vi "Data Retrieve GUI.vi"(0 "File or Folder Path":path=path "C:/", 1 "Data Type":T3=enum."DAT", 2 "DAT header length":i32=11, 5 "offset":i32, 7 "length":i32=1, 11 "error in (no error)":errorcluster) -> (4 "A vs B":cluster{dbl[], dbl[]}[](graph), 6 "C vs D":cluster{dbl[], dbl[]}[](graph), 8 "E":dbl[][](graph), 14 "Notes":string)   [LabVIEW 2019, in "LV-Data.lvclass"]
uses:
  LV-Data.lvclass
  <vilib>/Utility/miscctls.llb/LVOffsetAndMultiplierTypeDef.ctl
  LV-Data.ITX/Typedefs/Retrieve Data Type.ctl
  Typedefs/Map Variant--map.ctl
  b9190c8c-04b9-4fe6-9890-9f3313ef96ba.vi
  59021a08-4f23-4d52-b62b-93f2ba281558.vi
  LV-Data.ITX/LV-Data.ITX.lvclass
  <userlib>/LevyLab/Graph Utilities/graph_utilities.lvclass
panel:
  out "Current State":string
  in  "Update Graphs":bool
  in  "Read Files":bool
  in  "Initialize Keys":bool
  out "N":T1(array[cluster]) {"N5" format="%#_6p"; "N4" format="%#_6p"; "N3" format="%#_6p"; "N2" format="%#_6p"; "N1" format="%#_6p"}
  in  "keys":T2 {"N5" items=["AI1", "AI10", "AI11", "AI12", "AI2", "AI3", "AI4", "AI5", "AI6", "AI7", "AI8", "AI9", "AO1", "AO10", "AO11", "AO12", "AO2", "AO3", "AO4", "AO5", "AO6", "AO7", "AO8", "AO9", "Magnet", "Magnet Field", "OFF", "Temperature", "Time", "X1", "X10", "X11", "X12", "X2", "X3", "X4", "X5", "X6", "X7", "X8", "X9", "Y1", "Y10", "Y11", "Y12", "Y2", "Y3", "Y4", "Y5", "Y6", "Y7", "Y8", "Y9"]; "N4" items=["AI1", "AI10", "AI11", "AI12", "AI2", "AI3", "AI4", "AI5", "AI6", "AI7", "AI8", "AI9", "AO1", "AO10", "AO11", "AO12", "AO2", "AO3", "AO4", "AO5", "AO6", "AO7", "AO8", "AO9", "Magnet", "Magnet Field", "OFF", "Temperature", "Time", "X1", "X10", "X11", "X12", "X2", "X3", "X4", "X5", "X6", "X7", "X8", "X9", "Y1", "Y10", "Y11", "Y12", "Y2", "Y3", "Y4", "Y5", "Y6", "Y7", "Y8", "Y9"]; "N3" items=["AI1", "AI10", "AI11", "AI12", "AI2", "AI3", "AI4", "AI5", "AI6", "AI7", "AI8", "AI9", "AO1", "AO10", "AO11", "AO12", "AO2", "AO3", "AO4", "AO5", "AO6", "AO7", "AO8", "AO9", "Magnet", "Magnet Field", "OFF", "Temperature", "Time", "X1", "X10", "X11", "X12", "X2", "X3", "X4", "X5", "X6", "X7", "X8", "X9", "Y1", "Y10", "Y11", "Y12", "Y2", "Y3", "Y4", "Y5", "Y6", "Y7", "Y8", "Y9"]; "N2" items=["AI1", "AI10", "AI11", "AI12", "AI2", "AI3", "AI4", "AI5", "AI6", "AI7", "AI8", "AI9", "AO1", "AO10", "AO11", "AO12", "AO2", "AO3", "AO4", "AO5", "AO6", "AO7", "AO8", "AO9", "Magnet", "Magnet Field", "OFF", "Temperature", "Time", "X1", "X10", "X11", "X12", "X2", "X3", "X4", "X5", "X6", "X7", "X8", "X9", "Y1", "Y10", "Y11", "Y12", "Y2", "Y3", "Y4", "Y5", "Y6", "Y7", "Y8", "Y9"]; "N1" items=["AI1", "AI10", "AI11", "AI12", "AI2", "AI3", "AI4", "AI5", "AI6", "AI7", "AI8", "AI9", "AO1", "AO10", "AO11", "AO12", "AO2", "AO3", "AO4", "AO5", "AO6", "AO7", "AO8", "AO9", "Magnet", "Magnet Field", "OFF", "Temperature", "Time", "X1", "X10", "X11", "X12", "X2", "X3", "X4", "X5", "X6", "X7", "X8", "X9", "Y1", "Y10", "Y11", "Y12", "Y2", "Y3", "Y4", "Y5", "Y6", "Y7", "Y8", "Y9"]; "E" items=["AI1", "AI10", "AI11", "AI12", "AI2", "AI3", "AI4", "AI5", "AI6", "AI7", "AI8", "AI9", "AO1", "AO10", "AO11", "AO12", "AO2", "AO3", "AO4", "AO5", "AO6", "AO7", "AO8", "AO9", "Magnet", "Magnet Field", "OFF", "Temperature", "Time", "X1", "X10", "X11", "X12", "X2", "X3", "X4", "X5", "X6", "X7", "X8", "X9", "Y1", "Y10", "Y11", "Y12", "Y2", "Y3", "Y4", "Y5", "Y6", "Y7", "Y8", "Y9"]; "D" items=["AI1", "AI10", "AI11", "AI12", "AI2", "AI3", "AI4", "AI5", "AI6", "AI7", "AI8", "AI9", "AO1", "AO10", "AO11", "AO12", "AO2", "AO3", "AO4", "AO5", "AO6", "AO7", "AO8", "AO9", "Magnet", "Magnet Field", "OFF", "Temperature", "Time", "X1", "X10", "X11", "X12", "X2", "X3", "X4", "X5", "X6", "X7", "X8", "X9", "Y1", "Y10", "Y11", "Y12", "Y2", "Y3", "Y4", "Y5", "Y6", "Y7", "Y8", "Y9"]; "C" items=["AI1", "AI10", "AI11", "AI12", "AI2", "AI3", "AI4", "AI5", "AI6", "AI7", "AI8", "AI9", "AO1", "AO10", "AO11", "AO12", "AO2", "AO3", "AO4", "AO5", "AO6", "AO7", "AO8", "AO9", "Magnet", "Magnet Field", "OFF", "Temperature", "Time", "X1", "X10", "X11", "X12", "X2", "X3", "X4", "X5", "X6", "X7", "X8", "X9", "Y1", "Y10", "Y11", "Y12", "Y2", "Y3", "Y4", "Y5", "Y6", "Y7", "Y8", "Y9"]; "B" items=["AI1", "AI10", "AI11", "AI12", "AI2", "AI3", "AI4", "AI5", "AI6", "AI7", "AI8", "AI9", "AO1", "AO10", "AO11", "AO12", "AO2", "AO3", "AO4", "AO5", "AO6", "AO7", "AO8", "AO9", "Magnet", "Magnet Field", "OFF", "Temperature", "Time", "X1", "X10", "X11", "X12", "X2", "X3", "X4", "X5", "X6", "X7", "X8", "X9", "Y1", "Y10", "Y11", "Y12", "Y2", "Y3", "Y4", "Y5", "Y6", "Y7", "Y8", "Y9"]; "A" items=["AI1", "AI10", "AI11", "AI12", "AI2", "AI3", "AI4", "AI5", "AI6", "AI7", "AI8", "AI9", "AO1", "AO10", "AO11", "AO12", "AO2", "AO3", "AO4", "AO5", "AO6", "AO7", "AO8", "AO9", "Magnet", "Magnet Field", "OFF", "Temperature", "Time", "X1", "X10", "X11", "X12", "X2", "X3", "X4", "X5", "X6", "X7", "X8", "X9", "Y1", "Y10", "Y11", "Y12", "Y2", "Y3", "Y4", "Y5", "Y6", "Y7", "Y8", "Y9"]}
  in  "OK":bool
  in  "D  is time?":bool
  in  "B is time?":bool
  out "time":string[][](table)
  in  "Use Folder Index File?":bool
  in  "Generate Folder Index File?":bool
  in  "Ez name":string="Ez name"
  in  "Ey name":string="Ey name"
  in  "Ex name":string="Ex name"
  in  "C y name":string="C y name"
  in  "D x name":string="D x name"
  in  "A y name":string="A y name"
  in  "B x name":string="B x name"
  out "Index, Wavenames":string[][](table)
  in  "recolor traces?":bool
  in  "Ex":T4={"Offset"=0.0, "Multiplier"=1.0}
  in  "Ey":T4={"Offset"=0.0, "Multiplier"=1.0}
  out "counter":i32
  out "pattern":string="*.dat"
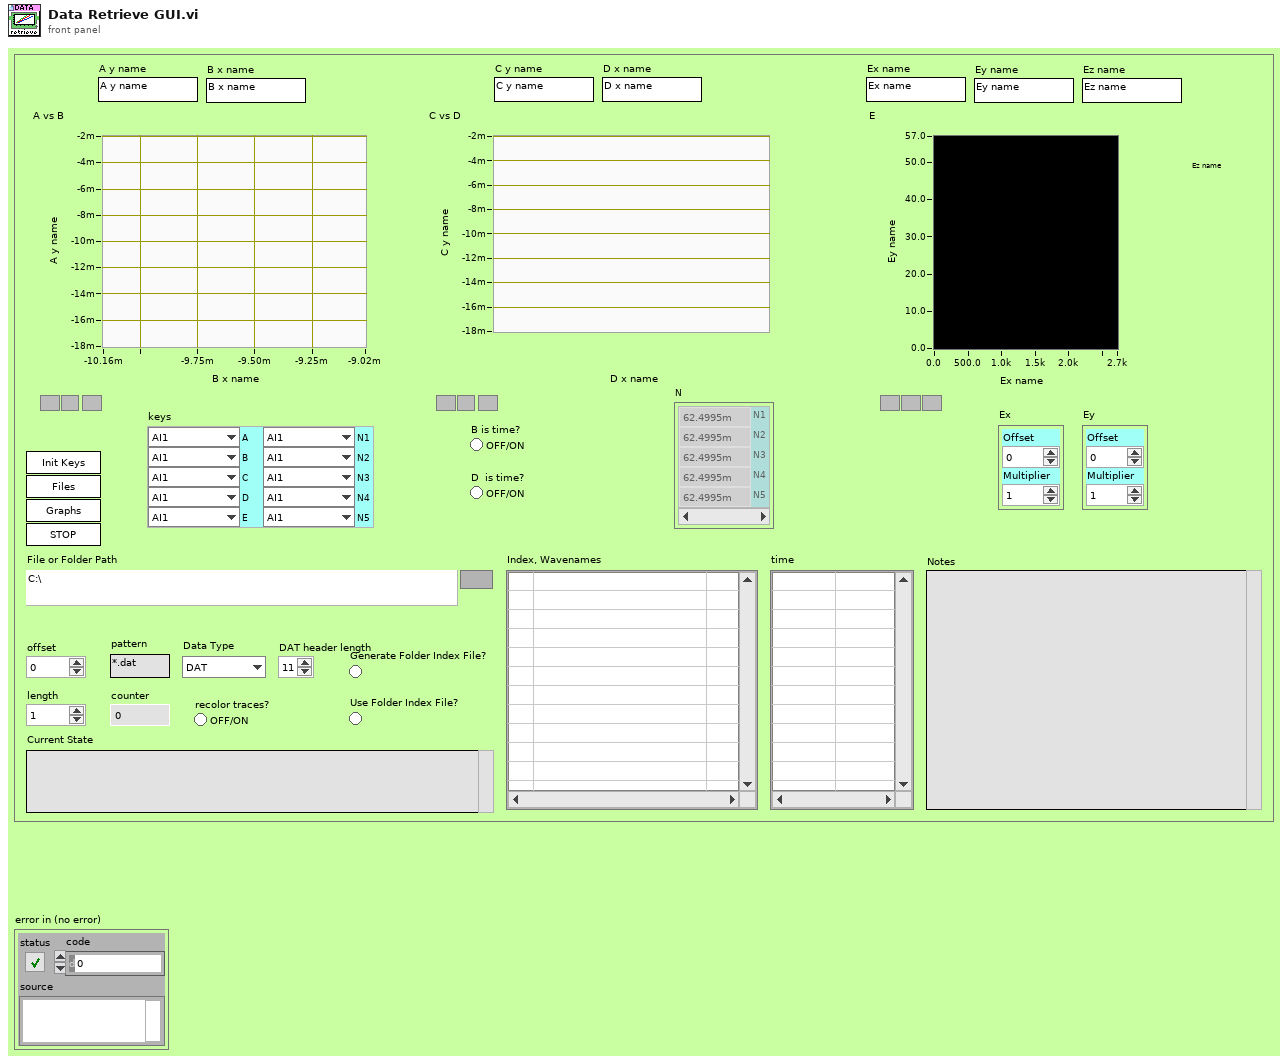
[diagram p1: front panel]
types:
  T1 = cluster{"N1":dbl, "N2":dbl, "N3":dbl, "N4":dbl, "N5":dbl}[]
  T2 = cluster{"A":u16, "B":u16, "C":u16, "D":u16, "E":u16, "N1":u16, "N2":u16, "N3":u16, "N4":u16, "N5":u16}
  T3 = typedef "LV-Data.ITX.lvclass/Retrieve Data Type.ctl" = enum16{"ITX", "ITX w/ 2D", "DAT", "TDMS"}
  T4 = typedef "LVOffsetAndMultiplierTypeDef.ctl" = cluster{"Offset":dbl, "Multiplier":dbl}
  T5 = enum32{"Invalid", "Standard", "Closed", "Hidden", "Minimized", "Maximized"}
  T6 = enum32{"invalid app kind", "Development System", "Run Time System", "Student Edition", "Embedded LabVIEW", "Evaluation", "Custom"}
  T7 = typedef "LV-Data.lvclass/Map Variant--map.ctl" = map{string, variant}
  T8 = cluster{"N1":dbl, "N2":dbl, "N3":dbl, "N4":dbl, "N5":dbl}
  T9 = cluster{"Core":cluster{"Current VI Reference":refnum<vi>, "Close Panel on Exit?":bool}, "Files":path[], "Append Index":i32, "Running Step":i32, "Data Map":T7[], "ring map":map{string, refnum<vi>}, "Wavenames":string[], "A vs B":cluster{dbl[], dbl[]}[], "C vs D":cluster{dbl[], dbl[]}[], "E":dbl[][]}
  T10 = cluster{"Current VI Reference":refnum<vi>, "Close Panel on Exit?":bool}
  T11 = typedef "LV-Data.lvclass/Dictionary--cluster.ctl" = cluster{"key":string, "value":variant}
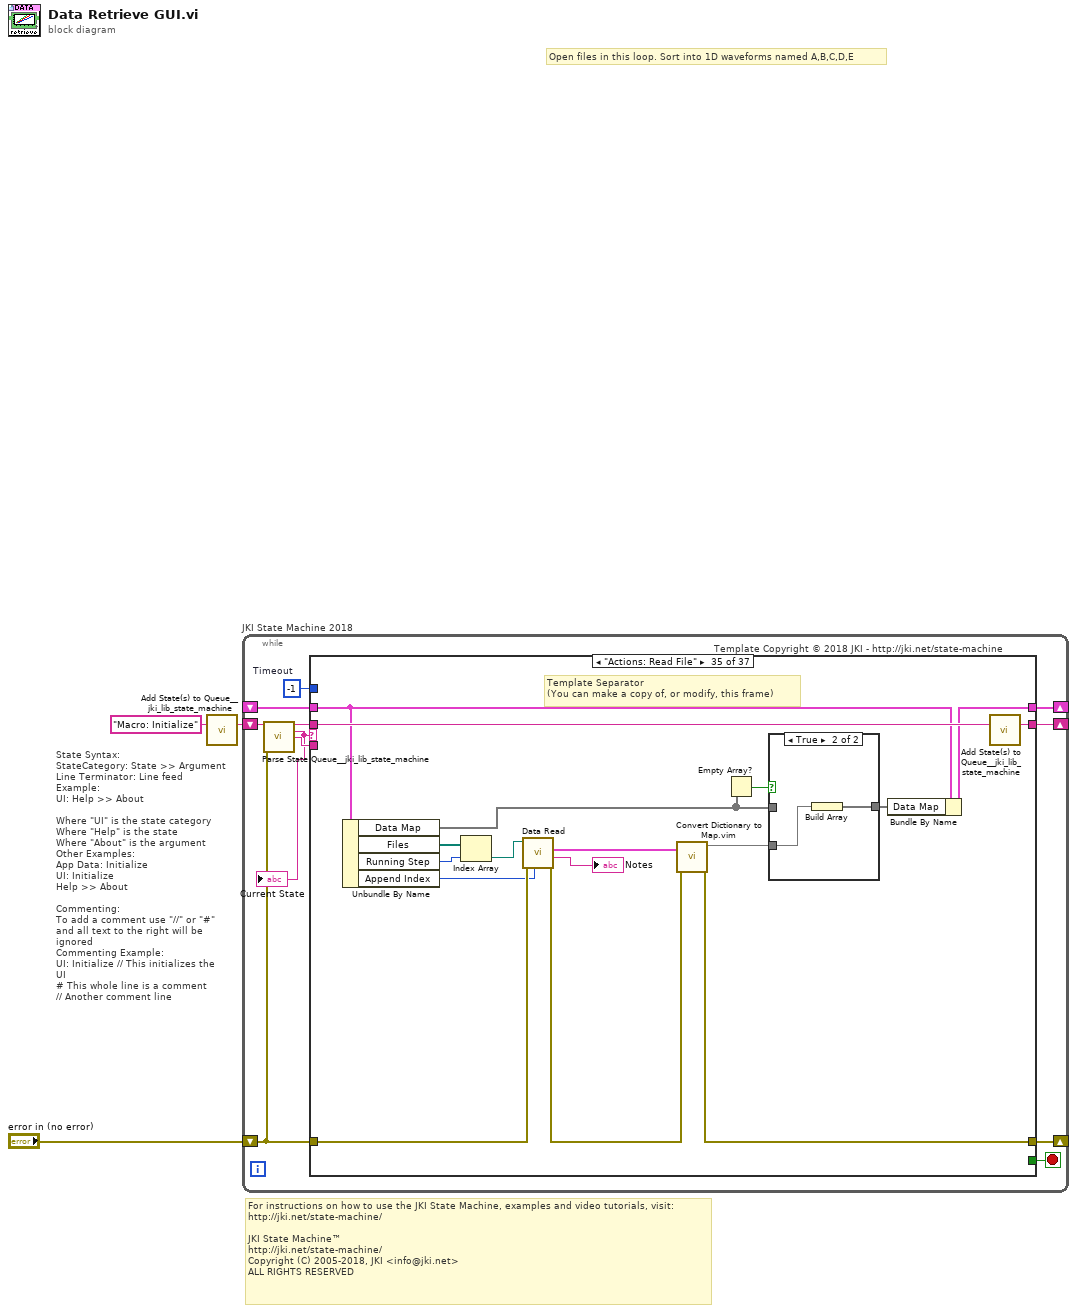
[diagram p0: block diagram]
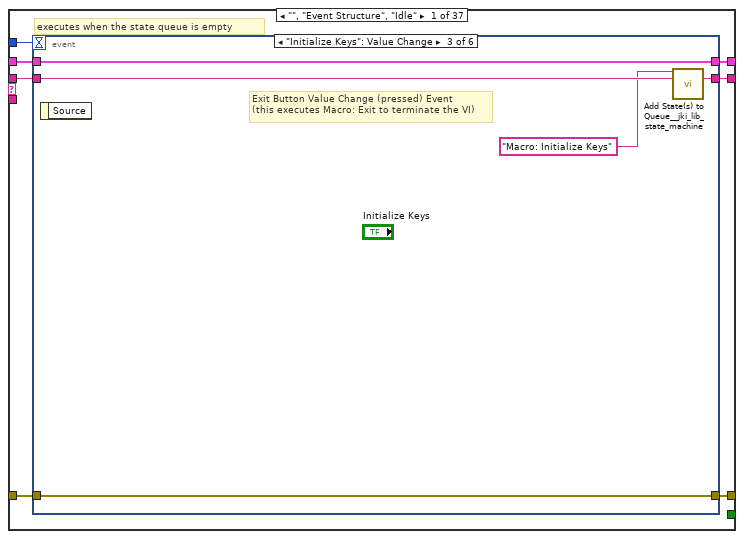
[diagram p2: hidden frame]
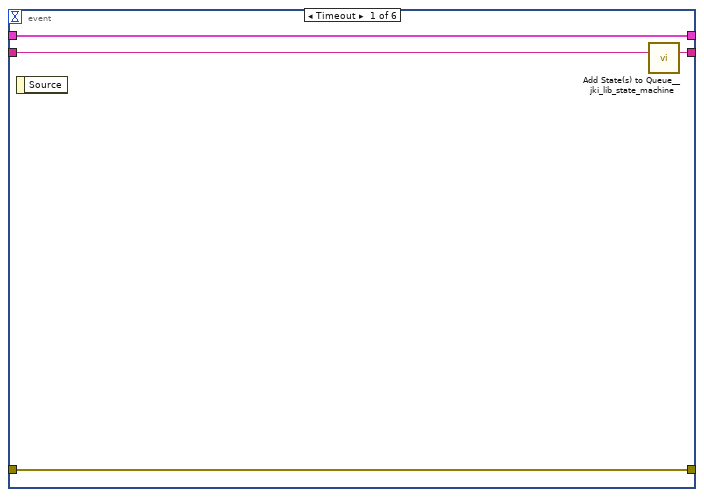
[diagram p3: hidden frame]
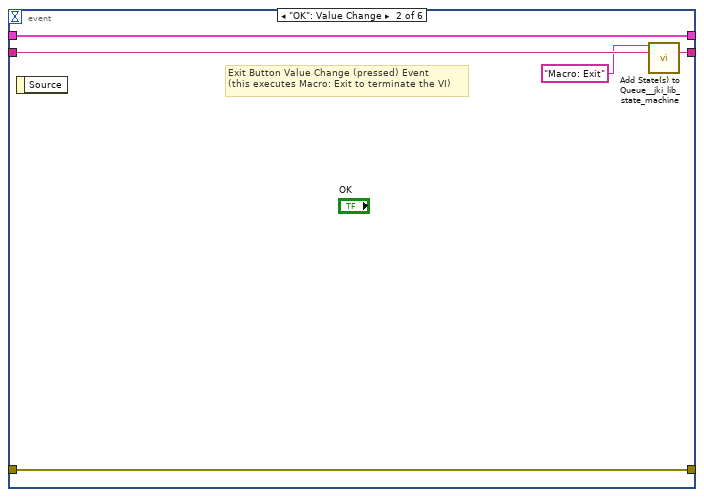
[diagram p4: hidden frame]
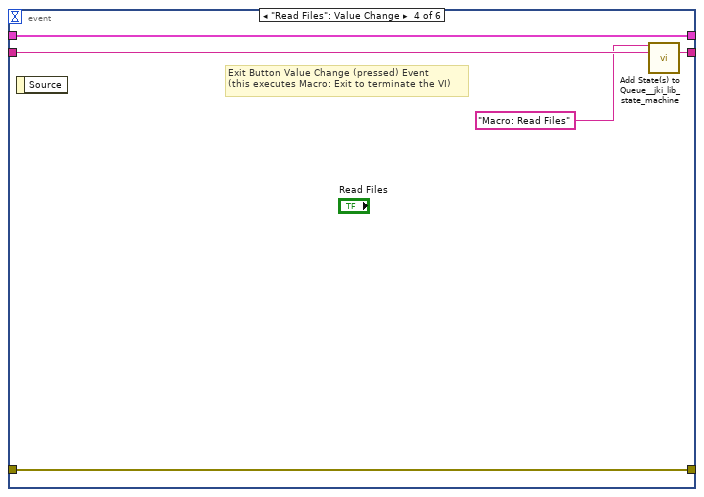
[diagram p5: hidden frame]
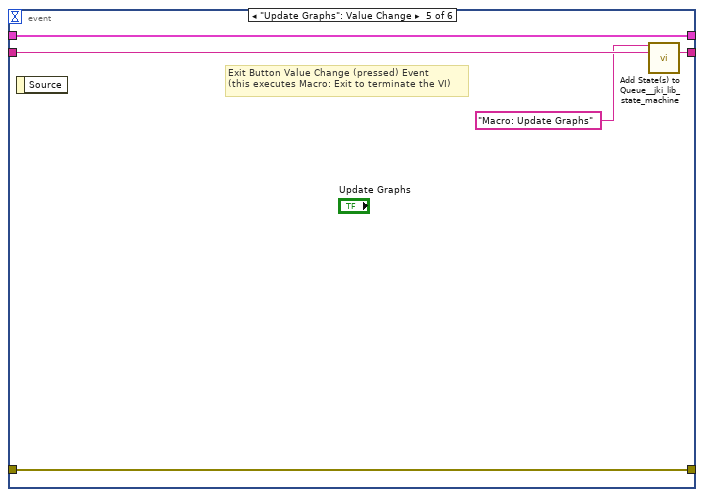
[diagram p6: hidden frame]
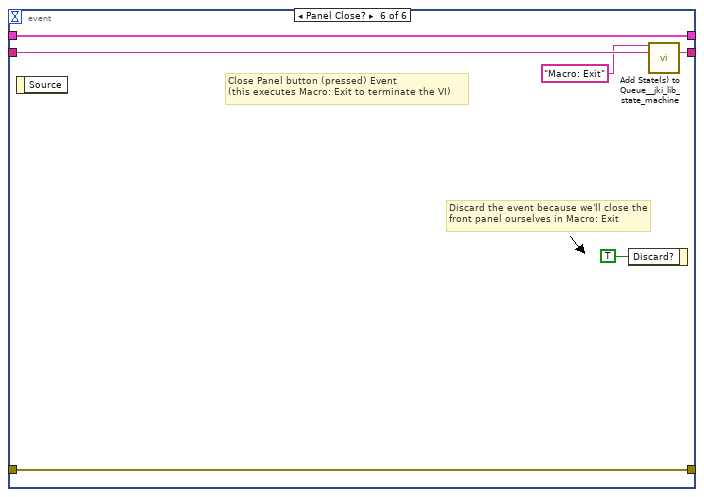
[diagram p7: hidden frame]
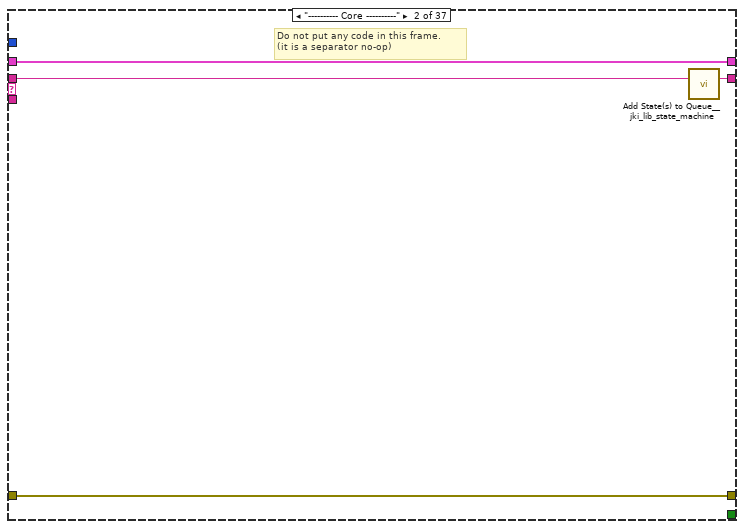
[diagram p8: hidden frame]
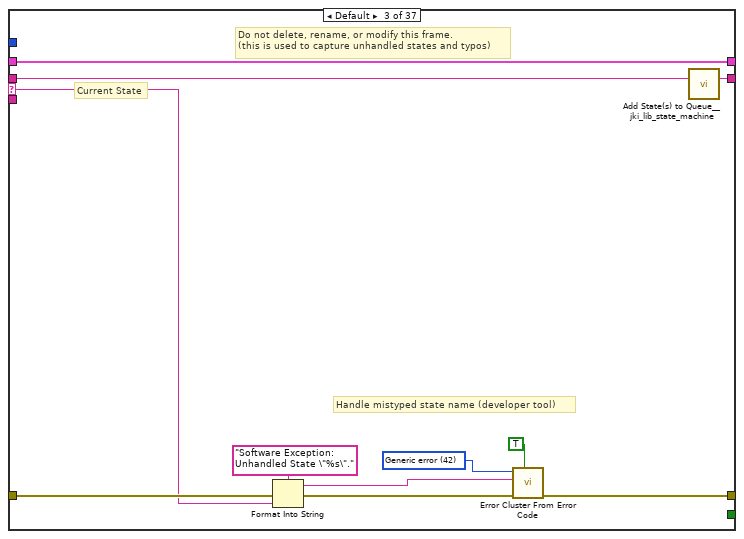
[diagram p9: hidden frame]
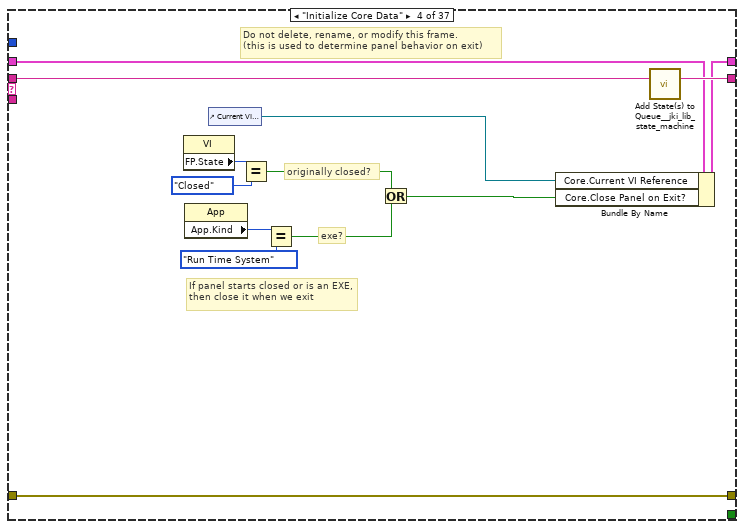
[diagram p10: hidden frame]
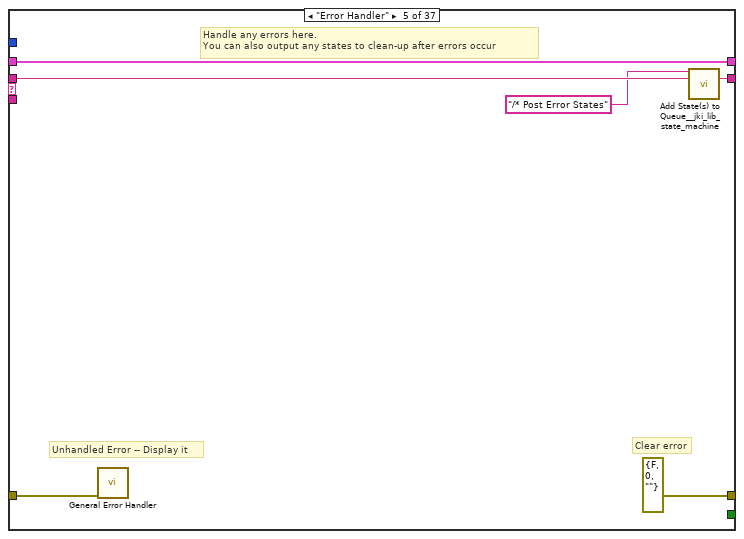
[diagram p11: hidden frame]
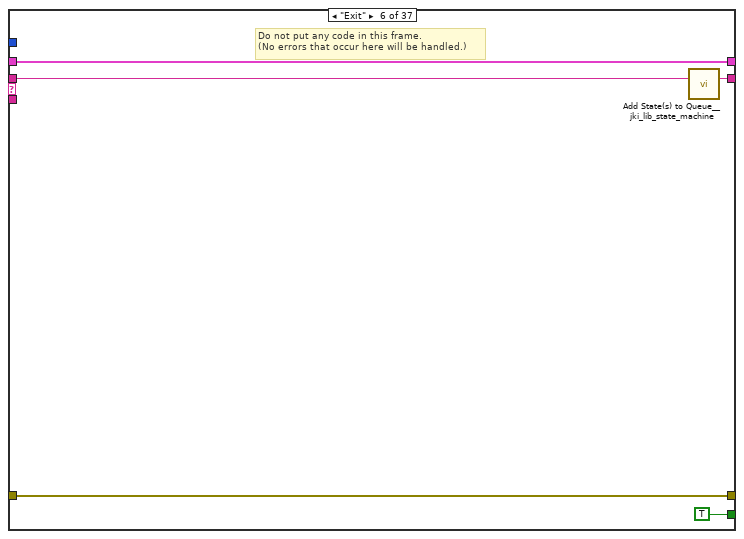
[diagram p12: hidden frame]
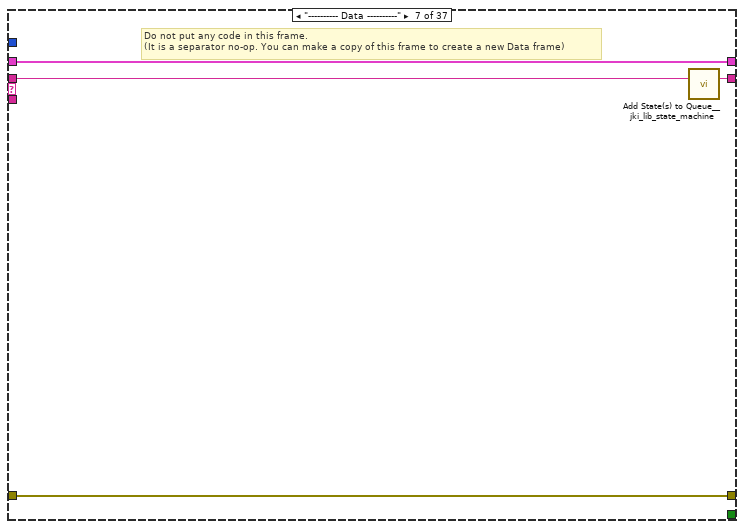
[diagram p13: hidden frame]
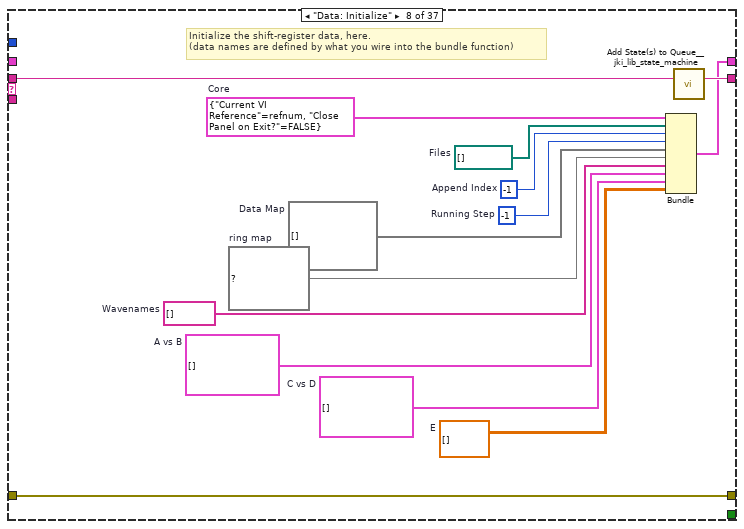
[diagram p14: hidden frame]
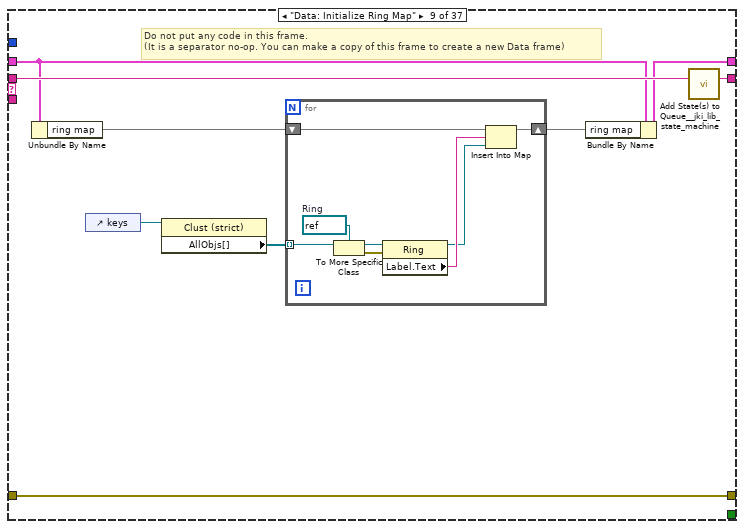
[diagram p15: hidden frame]
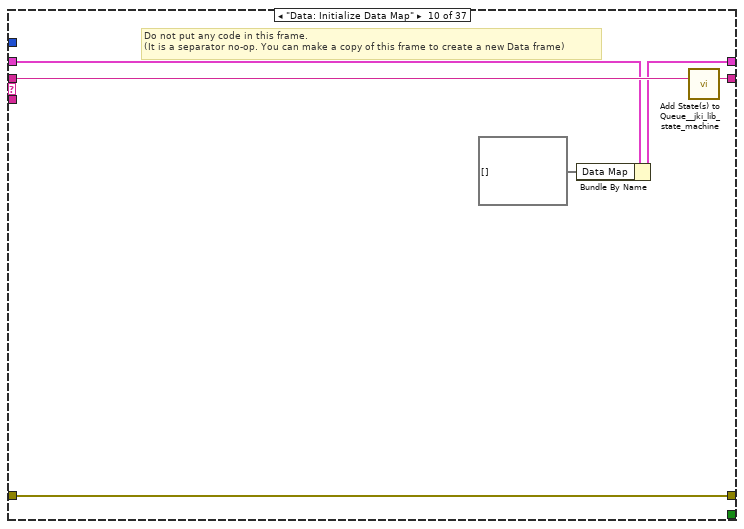
[diagram p16: hidden frame]
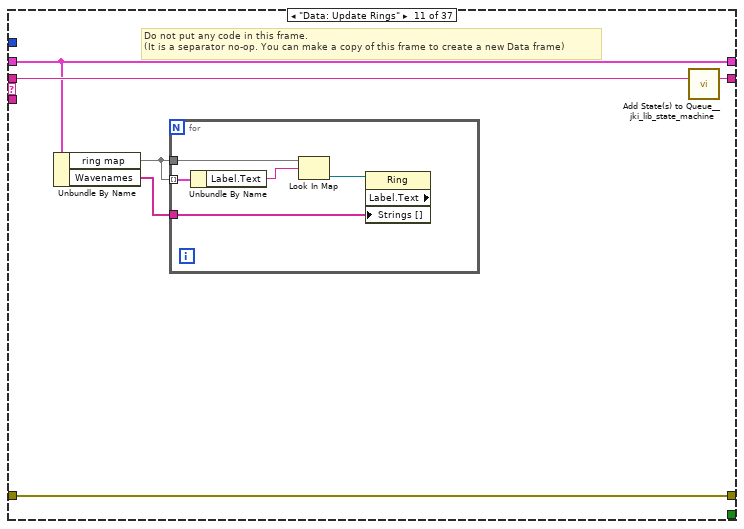
[diagram p17: hidden frame]
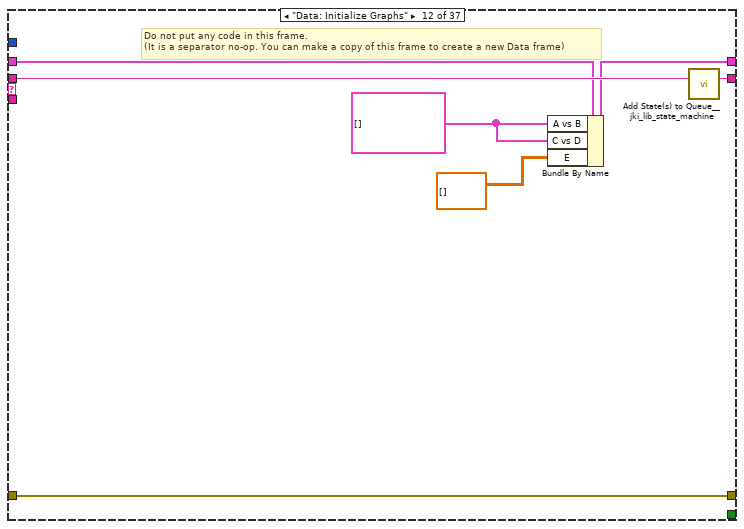
[diagram p18: hidden frame]
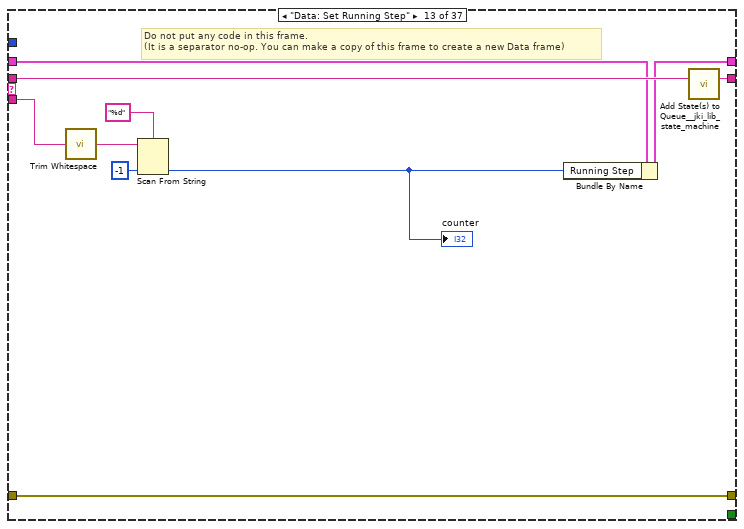
[diagram p19: hidden frame]
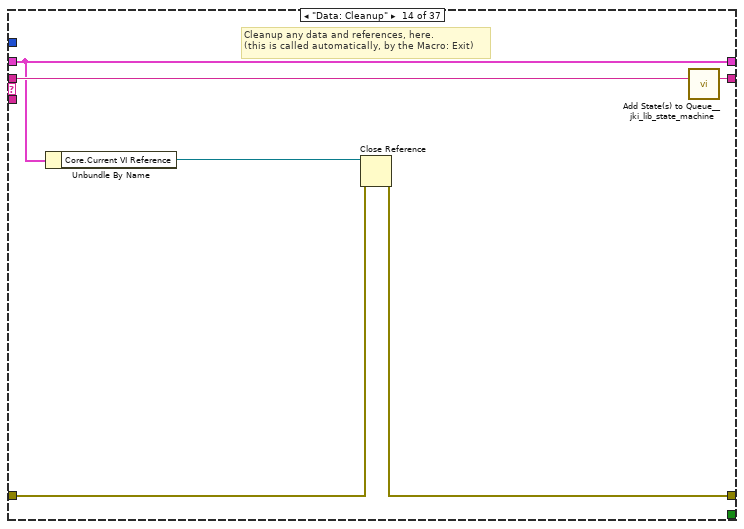
[diagram p20: hidden frame]
diagram:
  # "For instructions on how to use the JKI State Machine, examples and video tutorials, visit:\nhttp://jki.net/state-machine/\n\nJKI State Machine™\nhttp://jki.net/state-machine/\nCopyright (C) 2005-2018, JKI <info@jki.net>\nALL RIGHTS RESERVED"
  # "State Syntax:\nStateCategory: State >> Argument\nLine Terminator: Line feed\nExample:\nUI: Help >> About\n\nWhere \"UI\" is the state category\nWhere \"Help\" is the state\nWhere \"About\" is the argument\nOther Examples:\nApp Data: Initialize\nUI: Initialize\nHelp >> About\n\nCommenting:\nTo add a comment use \"//\" or \"#\" and all text to the right will be ignored\nCommenting Example:\nUI: Initialize // This initializes the UI\n# This whole line is a comment\n// Another comment line"
  # "Open files in this loop. Sort into 1D waveforms named A,B,C,D,E"
  n1 = call <vilib>:"Add State(s) to Queue__jki_lib_state_machine.vi"("State(s) in (\"\")"="Macro: Initialize") -> ("States Out"=w3:string)  [unwired: 14 in]
  n2 = while "JKI State Machine 2018" {
    shift-right: [w8] -> _
    shift-left: _ -> [w7]
    shift-right: [w11] -> _
    shift-left: "error in (no error)" -> [w5]
    shift-right: [w10] -> _
    shift-left: w3 -> [w12]
    stop <- w9 stop-if-true
    w6 = -1  # Timeout
    # "Template Copyright © 2018 JKI - http://jki.net/state-machine"
    n3 = call <vilib>:"Parse State Queue__jki_lib_state_machine.vi"("State Queue"=w12, "Error In (no error)"=w5) -> ("Remaining States"=w14:string, "Current State"=w4:string, "Arguments"=w13:string)  [unwired: 11 in]
    "Current State" <- w4
    n4 = case shown="\"Actions: Read File\"" w4 {
      selector: w4 -> [_ _ w56 _ _ _ _ _ _ _ _ _ _ _ _ _ _ _ _ _ _ _ _ _ _ _ _ _ _ _ _ _ _ _ _ _ _]
      tunnel: w14 -> [w21 w55 w60 w79 w85 w90 w94 w108 w117 w131 w137 w149 w159 w165 w169 w175 w181 w193 w199 w227 w234 w303 w308 w313 w328 w333 w338 w343 w348 w358 w362 w376 w423 w445 w464 w498 w519]
      tunnel: w13 -> [_ _ _ _ _ _ _ _ _ _ _ _ w154 _ _ _ w176 _ _ _ w228 _ _ _ w318 _ _ _ _ _ _ _ _ _ _ _ _]
      tunnel: w7 -> [w19 w52 w58 w72 w82 w88 w91 _ w109 w127 w134 w145 w155 w160 w166 w173 w179 w190 w195 w224 w230 w300 w305 w310 w325 w330 w335 w340 w345 w355 w359 w365 w418 w438 w453 w470 w516]
      tunnel: [w18 w53 w62 w76 errorcluster {"status"=FALSE, "code"=0, "source"=""} ("error out") w87 w92 w105 w115 w129 w135 w147 w157 w161 w167 w171 w177 w191 w197 w225 w231 w301 w306 w311 w326 w331 w336 w341 w346 w356 w360 w369 w421 w441 w455 w496 w517] -> w11
      tunnel: w5 -> [w17 w53 w61 w76 w81 w87 w92 w105 w115 w129 w135 w147 w157 w162 w167 w170 w178 w191 w197 w225 w232 w301 w306 w311 w326 w331 w336 w341 w346 w356 w360 w368 w421 w440 w460 w496 w517]
      tunnel: [w20 w54 w59 w78 w84 w89 w93 w107 w116 w130 w136 w148 w158 w164 w168 w174 w180 w192 w198 w226 w233 w302 w307 w312 w327 w332 w337 w342 w347 w357 w361 w375 w422 w444 w463 w497 w518] -> w10
      tunnel: [_ _ _ _ _ TRUE _ _ _ _ _ _ _ _ _ _ _ _ _ _ _ _ _ _ _ _ _ _ _ _ _ _ _ _ _ _ _] -> w9
      tunnel: [w16 w52 w58 w77 w82 w88 w91 w106 w110 w128 w134 w146 w156 w160 w166 w173 w179 w190 w195 w224 w230 w300 w305 w310 w325 w330 w335 w340 w345 w355 w359 w366 w419 w439 w454 w471 w516] -> w8
      tunnel: w6 -> [w15 _ _ _ _ _ _ _ _ _ _ _ _ _ _ _ _ _ _ _ _ _ _ _ _ _ _ _ _ _ _ _ _ _ _ _ _]
      frame "", "Event Structure", "Idle" {
        # "executes when the state queue is empty"
        n5 = event shown="[2] \"Initialize Keys\": Value Change" {
          selector: _ -> [_ _ _ _ _ _]
          dyn-events: _ -> [_ _ _ _ _ _]
          timeout: w15 -> [_ _ _ _ _ _]
          tunnel: w21 -> [w25 w30 w35 w40 w45 w51]
          tunnel: [w24 w29 w34 w39 w44 w50] -> w20
          tunnel: w19 -> [w22 w27 w32 w37 w42 w48]
          tunnel: [w23 w28 w33 w38 w43 w49] -> w18
          tunnel: w17 -> [w23 w28 w33 w38 w43 w49]
          tunnel: [w22 w27 w32 w37 w42 w48] -> w16
          event Timeout {
            n6 = event-data() -> ()  [unwired: 1 in, 1 out]
            n7 = call <vilib>:"Add State(s) to Queue__jki_lib_state_machine.vi"("State(s) in (\"\")"=w25) -> ("States Out"=w24:string)  [unwired: 14 in]
          }
          event "OK": Value Change {
            # "Exit Button Value Change (pressed) Event\n(this executes Macro: Exit to terminate the VI)"
            n8 = event-data() -> ()  [unwired: 1 in, 1 out]
            n9 = call <vilib>:"Add State(s) to Queue__jki_lib_state_machine.vi"("State(s) in Front (\"\")"="Macro: Exit", "State(s) in (\"\")"=w30) -> ("States Out"=w29:string)  [unwired: 13 in]
          }
          event "Initialize Keys": Value Change {
            # "Exit Button Value Change (pressed) Event\n(this executes Macro: Exit to terminate the VI)"
            n10 = event-data() -> ()  [unwired: 1 in, 1 out]
            n11 = call <vilib>:"Add State(s) to Queue__jki_lib_state_machine.vi"("State(s) in Front (\"\")"="Macro: Initialize Keys", "State(s) in (\"\")"=w35) -> ("States Out"=w34:string)  [unwired: 13 in]
          }
          event "Read Files": Value Change {
            # "Exit Button Value Change (pressed) Event\n(this executes Macro: Exit to terminate the VI)"
            n12 = event-data() -> ()  [unwired: 1 in, 1 out]
            n13 = call <vilib>:"Add State(s) to Queue__jki_lib_state_machine.vi"("State(s) in Front (\"\")"="Macro: Read Files", "State(s) in (\"\")"=w40) -> ("States Out"=w39:string)  [unwired: 13 in]
          }
          event "Update Graphs": Value Change {
            # "Exit Button Value Change (pressed) Event\n(this executes Macro: Exit to terminate the VI)"
            n14 = event-data() -> ()  [unwired: 1 in, 1 out]
            n15 = call <vilib>:"Add State(s) to Queue__jki_lib_state_machine.vi"("State(s) in Front (\"\")"="Macro: Update Graphs", "State(s) in (\"\")"=w45) -> ("States Out"=w44:string)  [unwired: 13 in]
          }
          event Panel Close? {
            # "Discard the event because we'll close the front panel ourselves in Macro: Exit"
            # "Close Panel button (pressed) Event\n(this executes Macro: Exit to terminate the VI)"
            n16 = event-data() -> ()  [unwired: 1 in, 1 out]
            n17 = event-data("Discard?"=TRUE) -> ()  [unwired: 1 in, 1 out]
            n18 = call <vilib>:"Add State(s) to Queue__jki_lib_state_machine.vi"("State(s) in Front (\"\")"="Macro: Exit", "State(s) in (\"\")"=w51) -> ("States Out"=w50:string)  [unwired: 13 in]
          }
        }
      }
      frame "---------- Core ----------" {
        # "Do not put any code in this frame.\n(it is a separator no-op)"
        n19 = call <vilib>:"Add State(s) to Queue__jki_lib_state_machine.vi"("State(s) in (\"\")"=w55) -> ("States Out"=w54:string)  [unwired: 14 in]
      }
      frame Default {
        w65 = 42 items=["No error", "Argument error", "Memory is full", "Out of zone", "End of file", "File already open", "Generic file I/O error", "File not found", "File permission error", "Disk is full", "Duplicate path", "Too many files open", "System feature not enabled", "Resource file not found", "Cannot add resource", "Resource not found", "Image not found", "Image memory error", "Pen does not exist", "Config type invalid", "Config token not found", "Config parse error", "Config memory error", "Bad external code format", "Bad external code offset", "External code not present", "Null window", "Destroy window error", "Null menu", "Print aborted", "Bad print record", "Print driver error", "Windows error during printing", "Memory error during printing", "Print dialog error", "Generic print error", "Invalid device refnum", "Device not found", "Device parameter error", "Device unit error", "Cannot open device", "Device call aborted", "Generic error", "Cancelled by user", "Object ID too low", "Object ID too high", "Object not in heap", "Unknown heap", "Unknown object (invalid DefProc)", "Unknown object (DefProc not in table)", "Message out of range", "Invalid (null) method", "Unknown message", "Manager call not supported", "Bad address", "Network operation in progress", "Network operation timed out", "Connection is busy", "Network attribute not supported", "Network error", "Address in use", "System out of memory", "Connection aborted", "Connection refused", "Not connected", "Already connected", "Connection closed", "Initialization error (interapplication manager)", "Bad occurrence", "Wait on unbound occurrence handler", "Occurrence queue overflow", "Datalog type conflict", "Unused", "Unrecognized type (interapplication manager)", "Memory corrupt", "Failed to make temporary DLL", "Old CIN version", "Drag socket not found", "Failed to load drop-object", "Failed to register OLE object", "Failed to release OLE object", "Format specifier type mismatch", "Unknown format specifier", "Too few format specifiers", "Too many format specifiers", "Scan failed", "Newer CIN version", "Error converting to variant", "Runtime menu error", "Password tampered", "Variant attribute not found", "Incompatible variant data type", "Event data is not available", "Event Store is not present", "Occurrence is not found", "Event Queue is not created", "Event info is not available", "Refnum passed is NULL", "Error retrieving Class GUID", "Error retrieving CoClass GUID", "Error retrieving TypeLib GUID.", "Bad built application magic bytes.", "Specific driver is different from the specific driver associated with the Logical Name.", "There is no session opened to the class driver.", "Max Error", "MAX - Error with config objects", "MAX - Error loading configuration", "MAX - Group not supported"]
        # "Current State"
        # "Do not delete, rename, or modify this frame.\n(this is used to capture unhandled states and typos)"
        # "Handle mistyped state name (developer tool)"
        n20 = Format Into String(format string="Software Exception: Unhandled State \"%s\"." ("message"), error in=w61, w56) -> (resulting string=w64:string, error out=w63:errorcluster)  [unwired: 1 in]
        n21 = call <vilib>:"Error Cluster From Error Code.vi"("show call chain? (False)"=TRUE, "error in (no error)"=w63, "error message (\"\")"=w64, "error code (0)"=w65) -> ("error out"=w62:errorcluster)  [unwired: 5 in]
        n22 = call <vilib>:"Add State(s) to Queue__jki_lib_state_machine.vi"("State(s) in (\"\")"=w60) -> ("States Out"=w59:string)  [unwired: 14 in]
      }
      frame "Initialize Core Data" {
        # "Do not delete, rename, or modify this frame.\n(this is used to determine panel behavior on exit)"
        # "originally closed?"
        # "exe?"
        # "If panel starts closed or is an EXE, then close it when we exit"
        n23 = property class="VI"() -> ("FP.State"=w69:T5)  [unwired: 2 in, 2 out]
        n24 = property class="App"() -> ("App.Kind"=w75:T6)  [unwired: 2 in, 2 out]
        n25 = control-ref of="Current VI Reference"() -> (w70:refnum<vi>)
        n26 = Equal?(x=w69, y=T5."Closed" ("Front Panel Window:State")) -> (x = y?=w67:bool)
        n27 = Equal?(x=w75, y=T6."Run Time System" ("Application:Kind")) -> (x = y?=w73:bool)
        n28 = Or(x=w67, y=w73) -> (x .or. y?=w71:bool)
        n29 = Bundle By Name(cluster=w72, "Core.Current VI Reference"=w70, "Core.Close Panel on Exit?"=w71) -> (w77:T9)
        n30 = call <vilib>:"Add State(s) to Queue__jki_lib_state_machine.vi"("State(s) in (\"\")"=w79) -> ("States Out"=w78:string)  [unwired: 14 in]
      }
      frame "Error Handler" {
        # "Unhandled Error -- Display it"
        # "Handle any errors here.\nYou can also output any states to clean-up after errors occur"
        # "Clear error"
        n31 = call <vilib>:"General Error Handler.vi"("error in (no error)"=w81) -> ()  [unwired: 10 in, 5 out]
        n32 = call <vilib>:"Add State(s) to Queue__jki_lib_state_machine.vi"("State(s) in Front (\"\")"="/* Post Error States", "State(s) in (\"\")"=w85) -> ("States Out"=w84:string)  [unwired: 13 in]
      }
      frame "Exit" {
        # "Do not put any code in this frame.\n(No errors that occur here will be handled.)"
        n33 = call <vilib>:"Add State(s) to Queue__jki_lib_state_machine.vi"("State(s) in (\"\")"=w90) -> ("States Out"=w89:string)  [unwired: 14 in]
      }
      frame "---------- Data ----------" {
        # "Do not put any code in this frame.\n(It is a separator no-op. You can make a copy of this frame to create a new Data frame)"
        n34 = call <vilib>:"Add State(s) to Queue__jki_lib_state_machine.vi"("State(s) in (\"\")"=w94) -> ("States Out"=w93:string)  [unwired: 14 in]
      }
      frame "Data: Initialize" {
        w95 = dbl[][] []  # E
        w96 = cluster{dbl[], dbl[]}[] []  # C vs D
        w97 = cluster{dbl[], dbl[]}[] []  # A vs B
        w98 = string[] []  # Wavenames
        w99 = map{string, refnum<vi>} {}  # ring map
        w100 = T7[] []  # Data Map
        w101 = -1  # Running Step
        w102 = -1  # Append Index
        w103 = path[] []  # Files
        w104 = T10 {"Current VI Reference"=refnum, "Close Panel on Exit?"=FALSE}  # Core
        # "Initialize the shift-register data, here.\n(data names are defined by what you wire into the bundle function)"
        n35 = Bundle("Core"=w104, "Files"=w103, "Append Index"=w102, "Running Step"=w101, "Data Map"=w100, "ring map"=w99, "Wavenames"=w98, "A vs B"=w97, "C vs D"=w96, "E"=w95) -> (w106:T9)  [unwired: 1 in]
        n36 = call <vilib>:"Add State(s) to Queue__jki_lib_state_machine.vi"("State(s) in (\"\")"=w108) -> ("States Out"=w107:string)  [unwired: 14 in]
      }
      frame "Data: Initialize Ring Map" {
        # "Do not put any code in this frame.\n(It is a separator no-op. You can make a copy of this frame to create a new Data frame)"
        n37 = Unbundle By Name(w109) -> ("ring map"=w112:map{string, refnum<vi>})
        n38 = control-ref of="keys"() -> (w114:refnum<vi>)
        n39 = property class="Clust (strict)"(reference=w114) -> ("AllObjs[]"=w113:refnum<vi>[])  [unwired: 1 in, 2 out]
        n40 = for {
          tunnel: w113 -> [w124] mode=indexing
          shift-right: [w121] -> w111
          shift-left: w112 -> [w120]
          w125 = refnum<vi> refnum  # Ring
          n41 = To More Specific Class(target class=w125, reference=w124) -> (specific class reference=w123:refnum<vi>, error out=w119:errorcluster)  [unwired: 1 in]
          n42 = property class="Ring"(reference=w123, error in=w119) -> (reference out=w118:refnum<vi>, "Label.Text"=w122:string)  [unwired: 1 out]
          n43 = Insert Into Map(map in=w120, key=w122, value=w118) -> (map out=w121:map{string, refnum<vi>})  [unwired: 2 out]
        }
        n44 = Bundle By Name(cluster=w109, "ring map"=w111) -> (w110:T9)
        n45 = call <vilib>:"Add State(s) to Queue__jki_lib_state_machine.vi"("State(s) in (\"\")"=w117) -> ("States Out"=w116:string)  [unwired: 14 in]
      }
      frame "Data: Initialize Data Map" {
        # "Do not put any code in this frame.\n(It is a separator no-op. You can make a copy of this frame to create a new Data frame)"
        n46 = Bundle By Name(cluster=w127, "Data Map"=T7[] []) -> (w128:T9)
        n47 = call <vilib>:"Add State(s) to Queue__jki_lib_state_machine.vi"("State(s) in (\"\")"=w131) -> ("States Out"=w130:string)  [unwired: 14 in]
      }
      frame "Data: Update Rings" {
        # "Do not put any code in this frame.\n(It is a separator no-op. You can make a copy of this frame to create a new Data frame)"
        n48 = Unbundle By Name(w134) -> ("ring map"=w133:map{string, refnum<vi>}, "Wavenames"=w132:string[])
        n49 = for {
          tunnel: w133 -> [w142] mode=indexing
          tunnel: w133 -> [w141]
          tunnel: w132 -> [w138]
          n50 = Unbundle By Name(w142) -> ("Label.Text"=w140:string)
          n51 = Look In Map(map=w141, key=w140) -> (value=w139:refnum<vi>)  [unwired: 1 in, 1 out]
          n52 = property class="Ring" props=["Label", "Text", "Strings []"](reference=w139, "Strings []"=w138) -> ()  [unwired: 1 in, 3 out]
        }
        n53 = call <vilib>:"Add State(s) to Queue__jki_lib_state_machine.vi"("State(s) in (\"\")"=w137) -> ("States Out"=w136:string)  [unwired: 14 in]
      }
      frame "Data: Initialize Graphs" {
        w144 = cluster{dbl[], dbl[]}[] [] ("A vs B")
        # "Do not put any code in this frame.\n(It is a separator no-op. You can make a copy of this frame to create a new Data frame)"
        n54 = Bundle By Name(cluster=w145, "A vs B"=w144, "C vs D"=w144, "E"=dbl[][] []) -> (w146:T9)
        n55 = call <vilib>:"Add State(s) to Queue__jki_lib_state_machine.vi"("State(s) in (\"\")"=w149) -> ("States Out"=w148:string)  [unwired: 14 in]
      }
      frame "Data: Set Running Step" {
        # "Do not put any code in this frame.\n(It is a separator no-op. You can make a copy of this frame to create a new Data frame)"
        n56 = call <vilib>:"Trim Whitespace.vi"("string"=w154) -> ("trimmed string"=w153:string)  [unwired: 1 in]
        n57 = Scan From String(format string="%d", input string=w153, default 1=-1 ("default value 1")) -> (output 1=w150:i32)  [unwired: 2 in, 3 out]
        "counter" <- w150
        n58 = Bundle By Name(cluster=w155, "Running Step"=w150) -> (w156:T9)
        n59 = call <vilib>:"Add State(s) to Queue__jki_lib_state_machine.vi"("State(s) in (\"\")"=w159) -> ("States Out"=w158:string)  [unwired: 14 in]
      }
      frame "Data: Cleanup" {
        # "Cleanup any data and references, here.\n(this is called automatically, by the Macro: Exit)"
        n60 = Unbundle By Name(w160) -> ("Core.Current VI Reference"=w163:refnum<vi>)
        n61 = Close Reference(reference=w163, error in (no error)=w162) -> (error out=w161:errorcluster)
        n62 = call <vilib>:"Add State(s) to Queue__jki_lib_state_machine.vi"("State(s) in (\"\")"=w165) -> ("States Out"=w164:string)  [unwired: 14 in]
      }
      frame "---------- UI ----------" {
        # "Do not put any code in this frame.\n(It is a separator no-op. You can make a copy of this frame to create a new UI frame)"
        n63 = call <vilib>:"Add State(s) to Queue__jki_lib_state_machine.vi"("State(s) in (\"\")"=w169) -> ("States Out"=w168:string)  [unwired: 14 in]
      }
      frame "UI: Initialize" {
        # "Initialize the User Interface, here.\n(this is called automatically, by the Macro: Init)"
        n64 = call <userlib>:"Fit VI window to Largest Dec__ogtk.vi"("error in (no error)"=w170, "border spacing (2 px)"=0) -> ("error out"=w171:errorcluster)  [unwired: 4 in, 1 out]
        n65 = call <vilib>:"Add State(s) to Queue__jki_lib_state_machine.vi"("State(s) in (\"\")"=w175) -> ("States Out"=w174:string)  [unwired: 14 in]
      }
      frame "UI: Cursor Set" {
        # "Argument"
        # "Set and Unset Cursor Busy.\n(Usage: \"UI: Cursor Set >> Busy|Idle\")"
        n66 = case shown="\"Idle\", Default" w176 {
          tunnel: w178 -> [w183 w185]
          tunnel: [w182 w184] -> w177
          frame "Idle", Default {
            n67 = call <vilib>:"Unset Busy.vi"("error in (no error)"=w183) -> ("error out"=w182:errorcluster)  [unwired: 10 in]
          }
          frame "Busy" {
            n68 = call <vilib>:"Set Busy.vi"("error in (no error)"=w185) -> ("error out"=w184:errorcluster)  [unwired: 9 in, 1 out]
          }
        }
        n69 = call <vilib>:"Add State(s) to Queue__jki_lib_state_machine.vi"("State(s) in (\"\")"=w181) -> ("States Out"=w180:string)  [unwired: 14 in]
      }
      frame "UI: Update Graphs" {
        # "Do not put any code in this frame.\n(It is a separator no-op. You can make a copy of this frame to create a new UI frame)"
        n70 = Unbundle By Name(w190) -> ("A vs B"=→"A vs B":cluster{dbl[], dbl[]}[], "C vs D"=→"C vs D":cluster{dbl[], dbl[]}[], "E"=w187:dbl[][])
        n71 = Transpose 2D Array(2D array=w187) -> (transposed array=→"E":dbl[][])
        n72 = call <vilib>:"Add State(s) to Queue__jki_lib_state_machine.vi"("State(s) in (\"\")"=w193) -> ("States Out"=w192:string)  [unwired: 14 in]
      }
      frame "UI: Recolor Graphs" {
        # "Template Separator\n(You can make a copy of, or modify, this frame)"
        n73 = Unbundle By Name(w195) -> ("A vs B"=w194:cluster{dbl[], dbl[]}[])
        n74 = case shown="True" "recolor traces?" {
          tunnel: w194 -> [_ w200]
          frame False {
          }
          frame True {
            n75 = Array Size(array=w200) -> (size(s)=w203:i32)
            n76 = call <userlib>:"Choose Color Table.vi"() -> ("Color Table"=w201:u32[])  [unwired: 8 in, 3 out]
            n77 = call <userlib>:"Choose Color Table.vi"("Size (256)"=w203) -> ("Color Table"=w202:u32[])  [unwired: 7 in, 3 out]
            n78 = for {
              tunnel: w202 -> [w204] mode=indexing
              i -> [w205]
              n79 = property on="A vs B" class="XYGraph (strict)"("Active Plot"=w205, "Plot.Plot Color"=w204) -> (error out=w206:errorcluster)  [unwired: 2 in, 1 out]
              n80 = property on="C vs D" class="XYGraph (strict)"(error in=w206, "Active Plot"=w205, "Plot.Plot Color"=w204, "Plot.Fill/Pt. Color"=w204) -> ()  [unwired: 1 in, 2 out]
            }
            n81 = property on="E" class="IntGraph (strict)"("Color Table"=w201) -> ()  [unwired: 2 in, 2 out]
          }
        }
        n82 = call <vilib>:"Add State(s) to Queue__jki_lib_state_machine.vi"("State(s) in (\"\")"=w199) -> ("States Out"=w198:string)  [unwired: 14 in]
      }
      frame "UI: Graph Labels" {
        # "Do not put any code in this frame.\n(It is a separator no-op. You can make a copy of this frame to create a new UI frame)"
        n83 = property on="E" class="IntGraph (strict)"("XScale.Ofst&Mult"="Ex", "YScale.Ofst&Mult"="Ey") -> ()  [unwired: 2 in, 2 out]
        n84 = property on="E" class="IntGraph (strict)"("XScale.NameLbl.Text"="Ex name", "YScale.NameLbl.Text"="Ey name", "ZScale.NameLbl.Text"="Ez name") -> ()  [unwired: 2 in, 2 out]
        n85 = Select(t=7.0, s="D  is time?", f=8.0) -> (s? t:f=w221:dbl)
        n86 = Select(t=7.0, s="B is time?", f=8.0) -> (s? t:f=w220:dbl)
        n87 = property on="A vs B" class="XYGraph (strict)"("XScale.Format"=w220, "XScale.NameLbl.Text"="B x name", "YScale.NameLbl.Text"="A y name") -> ()  [unwired: 2 in, 2 out]
        n88 = property on="C vs D" class="XYGraph (strict)"("XScale.Format"=w221, "XScale.NameLbl.Text"="D x name", "YScale.NameLbl.Text"="C y name") -> ()  [unwired: 2 in, 2 out]
        n89 = call <vilib>:"Add State(s) to Queue__jki_lib_state_machine.vi"("State(s) in (\"\")"=w227) -> ("States Out"=w226:string)  [unwired: 14 in]
      }
      frame "UI: Front Panel State" {
        # "Argument"
        # "Set Front Panel Open or Closed\n(Usage: \"UI: Front Panel State >> Open|Close\")"
        n90 = Unbundle By Name(w230) -> ("Core.Current VI Reference"=w229:refnum<vi>)
        n91 = case shown="\"Minimize\", \"Minimized\"" w228 {
          tunnel: w232 -> [w240 w255 w266 w279 w292]
          tunnel: [w242 w256 w268 w281 w294] -> w231
          tunnel: w229 -> [w241 w253 w267 w280 w293]
          frame "Open", "Standard", Default {
            w235 = T5."Standard" ("State")
            n92 = property class="VI"(reference=w241, error in=w240) -> (reference out=w238:refnum<vi>, error out=w239:errorcluster, "FP.State"=w237:T5)
            n93 = Not Equal?(x=w237, y=w235) -> (x != y?=w236:bool)
            n94 = case shown="True" w236 {
              tunnel: [w246 w248] -> w242
              tunnel: w239 -> [w245 w248]
              tunnel: w238 -> [w244 _]
              tunnel: w235 -> [w243 _]
              frame True {
                n95 = invoke class="VI" method="FP.Open"(reference=w244, error in=w245, "Activate"=TRUE, "State"=w243) -> (error out=w246:errorcluster)  [unwired: 1 in, 4 out]
              }
              frame False {
              }
            }
          }
          frame "Close", "Closed" {
            n96 = property class="VI"(reference=w253, error in=w255) -> (reference out=w252:refnum<vi>, error out=w254:errorcluster, "FP.State"=w250:T5)
            n97 = Not Equal?(x=w250, y=T5."Closed" ("Front Panel Window:State")) -> (x != y?=w249:bool)
            n98 = case shown="True" w249 {
              tunnel: [w257 w260] -> w256
              tunnel: w254 -> [w257 w259]
              tunnel: w252 -> [_ w258]
              frame False {
              }
              frame True {
                n99 = invoke class="VI" method="FP.Close"(reference=w258, error in=w259) -> (error out=w260:errorcluster)  [unwired: 1 in, 2 out]
              }
            }
          }
          frame "Hidden", "Hide" {
            w261 = T5."Hidden" ("State")
            n100 = property class="VI"(reference=w267, error in=w266) -> (reference out=w264:refnum<vi>, error out=w265:errorcluster, "FP.State"=w263:T5)
            n101 = Not Equal?(x=w263, y=w261) -> (x != y?=w262:bool)
            n102 = case shown="True" w262 {
              tunnel: [w272 w273] -> w268
              tunnel: w265 -> [w271 w273]
              tunnel: w264 -> [w270 _]
              tunnel: w261 -> [w269 _]
              frame True {
                n103 = invoke class="VI" method="FP.Open"(reference=w270, error in=w271, "State"=w269) -> (error out=w272:errorcluster)  [unwired: 2 in, 4 out]
              }
              frame False {
              }
            }
          }
          frame "Minimize", "Minimized" {
            w274 = T5."Minimized" ("State")
            n104 = property class="VI"(reference=w280, error in=w279) -> (reference out=w277:refnum<vi>, error out=w278:errorcluster, "FP.State"=w276:T5)
            n105 = Not Equal?(x=w276, y=w274) -> (x != y?=w275:bool)
            n106 = case shown="True" w275 {
              tunnel: [w285 w286] -> w281
              tunnel: w278 -> [w284 w286]
              tunnel: w277 -> [w283 _]
              tunnel: w274 -> [w282 _]
              frame True {
                n107 = invoke class="VI" method="FP.Open"(reference=w283, error in=w284, "State"=w282) -> (error out=w285:errorcluster)  [unwired: 2 in, 4 out]
              }
              frame False {
              }
            }
          }
          frame "Maximize", "Maximized" {
            w287 = T5."Maximized" ("State")
            n108 = property class="VI"(reference=w293, error in=w292) -> (reference out=w290:refnum<vi>, error out=w291:errorcluster, "FP.State"=w289:T5)
            n109 = Not Equal?(x=w289, y=w287) -> (x != y?=w288:bool)
            n110 = case shown="True" w288 {
              tunnel: [w298 w299] -> w294
              tunnel: w291 -> [w297 w299]
              tunnel: w290 -> [w296 _]
              tunnel: w287 -> [w295 _]
              frame True {
                n111 = invoke class="VI" method="FP.Open"(reference=w296, error in=w297, "State"=w295) -> (error out=w298:errorcluster)  [unwired: 2 in, 4 out]
              }
              frame False {
              }
            }
          }
        }
        n112 = call <vilib>:"Add State(s) to Queue__jki_lib_state_machine.vi"("State(s) in (\"\")"=w234) -> ("States Out"=w233:string)  [unwired: 14 in]
      }
      frame "---------- Macro ----------" {
        # "Do not put any code in this frame.\n(It is a separator no-op. You can make a copy of this frame to create a new Macro frame)"
        n113 = call <vilib>:"Add State(s) to Queue__jki_lib_state_machine.vi"("State(s) in (\"\")"=w303) -> ("States Out"=w302:string)  [unwired: 14 in]
      }
      frame "Macro: Initialize" {
        w304 = "Data: Initialize\nInitialize Core Data\nUI: Initialize\nUI: Front Panel State >> Open\nData: Initialize Ring Map"  # Data: Initialize Initialize Core Data UI: Initialize UI: Front Panel State >> Open Data: Initialize Ring Map
        # "Initialization Macro\n(This is called once, when the VI starts)"
        n114 = call <vilib>:"Add State(s) to Queue__jki_lib_state_machine.vi"("State(s) in Front (\"\")"=w304, "State(s) in (\"\")"=w308) -> ("States Out"=w307:string)  [unwired: 13 in]
      }
      frame "Macro: Initialize Keys" {
        # "Do not put any code in this frame.\n(It is a separator no-op. You can make a copy of this frame to create a new Macro frame)"
        n115 = call <vilib>:"Add State(s) to Queue__jki_lib_state_machine.vi"("State(s) in Front (\"\")"="Actions: List Folder\nActions: Folder Subset\nData: Set Running Step >> 0\nActions: Read File\nData: Set Running Step >> -1\nActions: List Keys\nData: Update Rings" ("State(s) in Front (\"\")"), "State(s) in (\"\")"=w313) -> ("States Out"=w312:string)  [unwired: 13 in]
      }
      frame "Macro: Run Sequence" {
        # "File\nGraph"
        # "Do not put any code in this frame.\n(It is a separator no-op. You can make a copy of this frame to create a new Macro frame)"
        n116 = Unbundle By Name(w325) -> ("Files"=w324:path[], "Running Step"=w315:i32)
        n117 = Array Size(array=w324) -> (size(s)=w317:i32)
        n118 = Decrement(x=w317) -> (x-1=w316:i32)
        n119 = Less?(x=w315, y=w316) -> (x < y?=w314:bool)
        n120 = Increment(x=w315) -> (x+1=w322:i32)
        n121 = Format Into String(format string="Data: Set Running Step >> %1$d\nMacro: %2$s Sequence\nMacro: Run Sequence >> %2$s", w322, w318) -> (resulting string=w320:string)  [unwired: 2 in, 1 out]
        n122 = Select(t=w320, s=w314, f="Data: Set Running Step >> -1") -> (s? t:f=w319:string)
        n123 = call <vilib>:"Add State(s) to Queue__jki_lib_state_machine.vi"("State(s) in Front (\"\")"=w319, "State(s) in (\"\")"=w328) -> ("States Out"=w327:string)  [unwired: 13 in]
      }
      frame "Macro: Read Files" {
        # "Do not put any code in this frame.\n(It is a separator no-op. You can make a copy of this frame to create a new Macro frame)"
        n124 = call <vilib>:"Add State(s) to Queue__jki_lib_state_machine.vi"("State(s) in Front (\"\")"="Macro: Initialize Keys\nMacro: Run Sequence >> File" ("State(s) in Front (\"\")"), "State(s) in (\"\")"=w333) -> ("States Out"=w332:string)  [unwired: 13 in]
      }
      frame "Macro: File Sequence" {
        # "Do not put any code in this frame.\n(It is a separator no-op. You can make a copy of this frame to create a new Macro frame)"
        n125 = call <vilib>:"Add State(s) to Queue__jki_lib_state_machine.vi"("State(s) in Front (\"\")"="Actions: Read File" ("State(s) in Front (\"\")"), "State(s) in (\"\")"=w338) -> ("States Out"=w337:string)  [unwired: 13 in]
      }
      frame "Macro: Update Graphs" {
        # "Do not put any code in this frame.\n(It is a separator no-op. You can make a copy of this frame to create a new Macro frame)"
        n126 = call <vilib>:"Add State(s) to Queue__jki_lib_state_machine.vi"("State(s) in Front (\"\")"="Data: Initialize Graphs\nUI: Graph Labels\nMacro: Run Sequence >> Graph\nUI: Recolor Graphs" ("State(s) in Front (\"\")"), "State(s) in (\"\")"=w343) -> ("States Out"=w342:string)  [unwired: 13 in]
      }
      frame "Macro: Graph Sequence" {
        # "Do not put any code in this frame.\n(It is a separator no-op. You can make a copy of this frame to create a new Macro frame)"
        n127 = call <vilib>:"Add State(s) to Queue__jki_lib_state_machine.vi"("State(s) in Front (\"\")"="Actions: Extract Data\nUI: Update Graphs" ("State(s) in Front (\"\")"), "State(s) in (\"\")"=w348) -> ("States Out"=w347:string)  [unwired: 13 in]
      }
      frame "Macro: Exit" {
        # "Exit Macro\n(This is called once, when the VI exits)"
        n128 = Unbundle By Name(w355) -> ("Core.Close Panel on Exit?"=w354:bool)
        n129 = Select(t="UI: Front Panel State >> Close", s=w354, f="") -> (s? t:f=w351:string)
        n130 = call <vilib>:"Add State(s) to Queue__jki_lib_state_machine.vi"("State(s) in (\"\")"=w351, "State(s) at Back (\"\")"="Data: Cleanup\nExit") -> ("States Out"=w349:string)  [unwired: 13 in]
        n131 = call <vilib>:"Add State(s) to Queue__jki_lib_state_machine.vi"("State(s) in Front (\"\")"=w349, "State(s) in (\"\")"=w358) -> ("States Out"=w357:string)  [unwired: 13 in]
      }
      frame "---------- Actions ----------" {
        # "Template Separator\n(You can make a copy of, or modify, this frame)"
        n132 = call <vilib>:"Add State(s) to Queue__jki_lib_state_machine.vi"("State(s) in (\"\")"=w362) -> ("States Out"=w361:string)  [unwired: 14 in]
      }
      frame "Actions: List Folder" {
        # "Folder Index is a way to store the list of files in a particular folder.\nSpeeds up execution next time you want to list the folder."
        # "if path = folder, return list of files according to filter.\notherwise return file name"
        # "List Folder.\n(List folder contents)"
        n133 = case shown="\"TDMS\"" "Data Type" {
          tunnel: ["*.itx" ("pattern") "*.dat" ("pattern") "*.tdms" ("pattern")] -> w363
          tunnel: "DAT header length" -> [_ w379 _]
          tunnel: [0 ("DAT header length") w379 0 ("DAT header length")] -> w364
          frame Default {
          }
          frame "DAT" {
          }
          frame "TDMS" {
          }
        }
        "pattern" <- w363
        n134 = case shown="False" "Use Folder Index File?" {
          tunnel: [w388 w409] -> w367
          tunnel: "File or Folder Path" -> [w390 w410]
          tunnel: "Generate Folder Index File?" -> [w383 _]
          tunnel: w363 -> [w387 _]
          tunnel: w368 -> [w386 w408]
          tunnel: [w384 w407] -> w369
          frame False {
            n135 = File/Directory Info(path=w390, error in=w386) -> (directory=w389:bool, error out=w385:errorcluster)  [unwired: 5 out]
            n136 = case shown="True" w389 {
              tunnel: [w393 w401] -> w388
              tunnel: w390 -> [w392 w395]
              tunnel: w383 -> [_ w394]
              tunnel: w387 -> [_ w400]
              tunnel: w385 -> [w391 w398]
              tunnel: [w391 w399] -> w384
              frame False {
                n137 = Build Array(w392) -> (w393:path[])
              }
              frame True {
                n138 = call <vilib>:"Recursive File List.vi"("pattern"=w400, "error in (no error)"=w398, "Folder Path"=w395) -> ("error out"=w397:errorcluster, "All Files in Dir"=w401:path[], "dup Folder Path"=w396:path)  [unwired: 4 in, 2 out]
                n139 = case shown="False" w394 {
                  tunnel: w401 -> [_ w406]
                  tunnel: w396 -> [_ w405]
                  tunnel: w397 -> [w402 w404]
                  tunnel: [w402 w403] -> w399
                  frame False {
                  }
                  frame True {
                    n140 = call "Create Folder Index.vi"("error in (no error)"=w404, "File or Folder Path"=w405, "All Files in Dir"=w406) -> ("error out"=w403:errorcluster)  [unwired: 8 in]
                  }
                }
              }
            }
          }
          frame True {
            n141 = call "Read Folder Index.vi"("error in (no error)"=w408, "File or Folder Path"=w410) -> ("error out"=w407:errorcluster, "Files"=w409:path[])  [unwired: 8 in]
          }
        }
        n142 = Bundle By Name(cluster=w365, "Files"=w367, "Append Index"=w364) -> (w366:T9)
        n143 = call <vilib>:"Add State(s) to Queue__jki_lib_state_machine.vi"("State(s) in (\"\")"=w376) -> ("States Out"=w375:string)  [unwired: 14 in]
      }
      frame "Actions: Folder Subset" {
        # "Action: Folder Subset.\n2. Subset of files)"
        n144 = Unbundle By Name(w418) -> ("Files"=w420:path[])
        n145 = Less Than 0?(x="offset") -> (x < 0?=w413:bool)
        n146 = Less Than 0?(x="length") -> (x < 0?=w412:bool)
        n147 = Or(x=w413, y=w412) -> (x .or. y?=w411:bool)
        n148 = case shown="False" w411 {
          tunnel: w420 -> [w427 w428]
          tunnel: [w424 w428] -> w417
          tunnel: "length" -> [w426 _]
          tunnel: "offset" -> [w425 _]
          frame False {
            n149 = Array Subset(array=w427, index=w425, length=w426) -> (w424:path[])
          }
          frame True {
          }
        }
        n150 = for {
          tunnel: w417 -> [w430] mode=indexing
          tunnel: [w429] -> w416 mode=indexing
          n151 = File/Directory Info(path=w430) -> (last mod=w431:timestamp)  [unwired: 1 in, 6 out]
          n152 = Get Date/Time String(seconds (now)=w431) -> (date string=w433:string, time string=w432:string)  [unwired: 2 in]
          n153 = Build Array(w433, w432) -> (w429:string[])
        }
        "time" <- w416
        n154 = Bundle By Name(cluster=w418, "Files"=w417) -> (w419:T9)
        n155 = call <vilib>:"Add State(s) to Queue__jki_lib_state_machine.vi"("State(s) in (\"\")"=w423) -> ("States Out"=w422:string)  [unwired: 14 in]
      }
      frame "Actions: List Keys" {
        # "Template Separator\n(You can make a copy of, or modify, this frame)"
        n156 = Unbundle By Name(w438) -> ("Data Map"=w443:T7[])
        n157 = Index Array(array=w443) -> (element=w442:T7)  [unwired: 1 in]
        n158 = call "List Map Keys and Values.vim"("error in (no error)"=w440, "map in"=w442) -> ("error out"=w441:errorcluster, "Keys"=w434:string[])  [unwired: 6 in, 2 out]
        n159 = for {
          tunnel: w434 -> [_] mode=indexing
          tunnel: [w446] -> w435 mode=indexing
          i -> [w447]
          n160 = Number To Decimal String(number=w447) -> (decimal integer string=w446:string)  [unwired: 1 in]
        }
        n161 = Bundle By Name(cluster=w438, "Wavenames"=w434) -> (w439:T9)
        n162 = Build Array(w435, w434) -> (w437:string[][])
        n163 = Transpose 2D Array(2D array=w437) -> (transposed array=→"Index, Wavenames":string[][])
        n164 = call <vilib>:"Add State(s) to Queue__jki_lib_state_machine.vi"("State(s) in (\"\")"=w445) -> ("States Out"=w444:string)  [unwired: 14 in]
      }
      frame "Actions: Read File" {
        # "Template Separator\n(You can make a copy of, or modify, this frame)"
        n165 = Unbundle By Name(w453) -> ("Data Map"=w448:T7[], "Files"=w462:path[], "Running Step"=w451:i32, "Append Index"=w459:i32)
        n166 = Index Array(array=w462, index=w451) -> (element=w461:path)
        n167 = call "Data Read.vi"("Append Index"=w459, "error in (no error)"=w460, "path"=w461) -> ("error out"=w456:errorcluster, "Notes"=→"Notes":string, "Data (Dictionary)"=w457:T11[])  [unwired: 5 in, 1 out]
        n168 = call "Convert Dictionary to Map.vim"("error in (no error)"=w456, "Data (Dictionary)"=w457) -> ("error out"=w455:errorcluster, "map out"=w449:T7)  [unwired: 8 in]
        n169 = Empty Array?(array=w448) -> (empty?=w450:bool)
        n170 = case shown="True" w450 {
          tunnel: [w466 w469] -> w452
          tunnel: w448 -> [w467 _]
          tunnel: w449 -> [w465 w468]
          frame False {
            n171 = Build Array (concatenate)(w467, w465) -> (w466:T7[])
          }
          frame True {
            n172 = Build Array(w468) -> (w469:T7[])
          }
        }
        n173 = Bundle By Name(cluster=w453, "Data Map"=w452) -> (w454:T9)
        n174 = call <vilib>:"Add State(s) to Queue__jki_lib_state_machine.vi"("State(s) in (\"\")"=w464) -> ("States Out"=w463:string)  [unwired: 14 in]
      }
      frame "Actions: Extract Data" {
        # "Template Separator\n(You can make a copy of, or modify, this frame)"
        n175 = Unbundle By Name(w470) -> ("A vs B"=w481:cluster{dbl[], dbl[]}[], "C vs D"=w477:cluster{dbl[], dbl[]}[], "E"=w473:dbl[][])
        n176 = Unbundle By Name(w470) -> ("Data Map"=w495:T7[], "Running Step"=w482:i32, "ring map"=w483:map{string, refnum<vi>})
        n177 = for {
          tunnel: w495 -> [w508]
          tunnel: w483 -> [w512]
          tunnel: string[] ["B", "A", "D", "C", "E", "N1", "N2", "N3", "N4", "N5"] ("key") -> [w513] mode=indexing
          tunnel: [w511] -> w479 mode=indexing
          tunnel: w482 -> [w507]
          # "each"
          n178 = Look In Map(map=w512, key=w513) -> (value=w515:refnum<vi>)  [unwired: 1 in, 1 out]
          n179 = property class="Ring"(reference=w515) -> ("RingText.Text"=w514:string)  [unwired: 1 in, 2 out]
          n180 = Index Array(array=w508, index=w507) -> (element=w506:T7)
          n181 = Look In Map(map=w506, key=w514) -> (value=w510:variant)  [unwired: 1 in, 1 out]
          n182 = Variant To Data(type=dbl[] [], Variant=w510) -> (data=w511:dbl[])  [unwired: 1 in, 1 out]
        }
        n183 = Index Array(array=w479) -> (element #1=w493:dbl[], element #2=w492:dbl[], element #3=w491:dbl[], element #4=w490:dbl[], element #5=w472:dbl[], element #6=w489:dbl[], element #7=w488:dbl[], element #8=w487:dbl[], element #9=w486:dbl[], element #10=w485:dbl[])  [unwired: 20 in]
        n184 = Bundle(w493, w492) -> (w480:cluster{dbl[], dbl[]})  [unwired: 1 in]
        n185 = Bundle(w491, w490) -> (w475:cluster{dbl[], dbl[]})  [unwired: 1 in]
        n186 = Build Array (concatenate)(w481, w480) -> (w478:cluster{dbl[], dbl[]}[])
        n187 = Build Array (concatenate)(w477, w475) -> (w476:cluster{dbl[], dbl[]}[])
        n188 = Build Array (concatenate)(w473, w472) -> (w474:dbl[][])
        n189 = for {
          tunnel: w489 -> [w504] mode=indexing
          tunnel: w488 -> [w503] mode=indexing
          tunnel: w487 -> [w502] mode=indexing
          tunnel: w486 -> [w501] mode=indexing
          tunnel: w485 -> [w500] mode=indexing
          tunnel: [w505] -> w484 mode=indexing
          n190 = Bundle By Name(cluster=T8 {"N1"=0.0, "N2"=0.0, "N3"=0.0, "N4"=0.0, "N5"=0.0} ("N"), "N1"=w504, "N2"=w503, "N3"=w502, "N4"=w501, "N5"=w500) -> (w505:T8)
        }
        "N" <- w484
        n191 = Bundle By Name(cluster=w470, "A vs B"=w478, "C vs D"=w476, "E"=w474) -> (w471:T9)
        n192 = call <vilib>:"Add State(s) to Queue__jki_lib_state_machine.vi"("State(s) in (\"\")"=w498) -> ("States Out"=w497:string)  [unwired: 14 in]
      }
      frame "---------- Graph ----------" {
        # "Template Separator\n(You can make a copy of, or modify, this frame)"
        n193 = call <vilib>:"Add State(s) to Queue__jki_lib_state_machine.vi"("State(s) in (\"\")"=w519) -> ("States Out"=w518:string)  [unwired: 14 in]
      }
    }
  }
